vi "VI_get_version.vi"(8 "error in (no error)":errorcluster, 11 "vers block":string) -> (0 "error out":errorcluster, 3 "Version":T1 {"Flags" format="%04x"})   [LabVIEW 2023]
uses:
  <vilib>/Utility/error.llb/Error Cluster From Error Code.vi
  <vilib>/ErrorRing/Error Ring.xnode
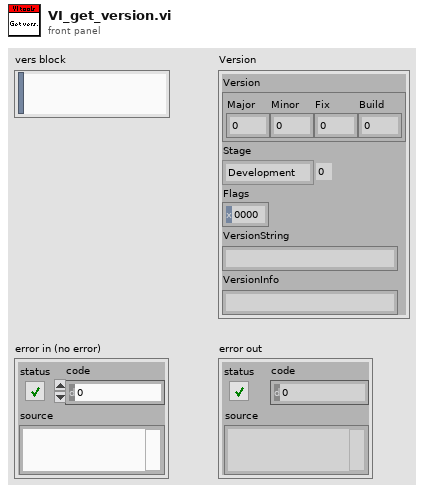
[diagram p1: front panel]
types:
  T1 = cluster{"Version":cluster{"Major":u8, "Minor":u8, "Fix":u8, "Build":u8}, "Stage":enum8{"Development", "Alpha", "Beta", "Release"}, "Flags":u16, "VersionString":string, "VersionInfo":string}
  T2 = cluster{"Version":u32, "Flags":u16, "VerStrLen":u8}
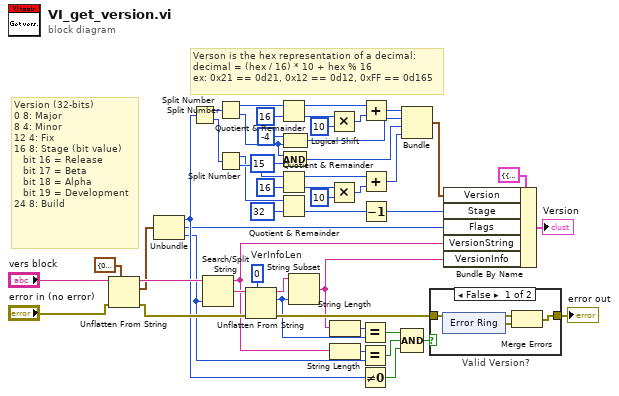
[diagram p0: block diagram]
diagram:
  w46 = u8 0  # VerInfoLen
  # "Verson is the hex representation of a decimal:\ndecimal = (hex / 16) * 10 + hex % 16\nex: 0x21 == 0d21, 0x12 == 0d12, 0xFF == 0d165"
  # "Version (32-bits)\n0 8: Major\n8 4: Minor\n12 4: Fix\n16 8: Stage (bit value)\n   bit 16 = Release\n   bit 17 = Beta\n   bit 18 = Alpha\n   bit 19 = Development\n24 8: Build"
  n1 = Unflatten From String(type=T2 {"Version"=0, "Flags"=0, "VerStrLen"=0} ("vers"), binary string="vers block", error in (no error)="error in (no error)") -> (rest of the binary string=w10:string, value=w4:T2, error out=w45:errorcluster)  [unwired: 2 in]
  n2 = Unbundle(w4) -> ("Version"=w3:u32, "Flags"=w2:u16, "VerStrLen"=w1:u8)
  n3 = Split Number(x=w3) -> (hi(x)=w42:u16, lo(x)=w43:u16)
  n4 = Search/Split String(string=w10, offset (0)=w1) -> (substring before match=w17:string, match + rest of string=w44:string)  [unwired: 1 in, 1 out]
  n5 = Split Number(x=w42) -> (hi(x)=w41:u8, lo(x)=w25:u8)
  n6 = Split Number(x=w43) -> (hi(x)=w21:u8, lo(x)=w30:u8)
  n7 = Unflatten From String(type=w46, binary string=w44, error in (no error)=w45) -> (rest of the binary string=w8:string, value=w9:u8, error out=w14:errorcluster)  [unwired: 2 in]
  n8 = Quotient & Remainder(x=w41, y=u8 16) -> (x-y*floor(x/y)=w36:u8, floor(x/y)=w39:u8)
  n9 = Quotient & Remainder(x=w30, y=u8 16) -> (x-y*floor(x/y)=w35:u8, floor(x/y)=w32:u8)
  n10 = Quotient & Remainder(x=w21, y=u8 32) -> (floor(x/y)=w20:u8)  [unwired: 1 out]
  n11 = Logical Shift(y=i16 -4, x=w25) -> (x << y=w23:u8)
  n12 = And(x=w25, y=u8 15) -> (x .and. y?=w26:u8)
  n13 = String Subset(string=w8, length (rest)=w9) -> (substring=w7:string)  [unwired: 1 in]
  n14 = Multiply(x=w39, y=u8 10) -> (x*y=w37:u8)
  n15 = Multiply(x=w32, y=u8 10) -> (x*y=w34:u8)
  n16 = String Length(string=w7) -> (length=w5:i32)
  n17 = String Length(string=w17) -> (length=w6:i32)
  n18 = Equal?(x=w5, y=w9) -> (x = y?=w16:bool)
  n19 = Equal?(x=w6, y=w1) -> (x = y?=w15:bool)
  n20 = Not Equal To 0?(x=w3) -> (x != 0?=w12:bool)
  n21 = Add(x=w36, y=w37) -> (x+y=w29:u8)
  n22 = Add(x=w35, y=w34) -> (x+y=w28:u8)
  n23 = Decrement(x=w20) -> (x-1=w18:u8)
  n24 = Compound Arithmetic op=AND(w16, w15, w12) -> (w13:bool)
  n25 = Bundle(w29, w23, w26, w28) -> (w19:cluster{u8, u8, u8, u8})  [unwired: 1 in]
  n26 = case "Valid Version?" shown="False" w13 {
    tunnel: [w53 w60] -> w49
    tunnel: w14 -> [w54 w60]
    frame False {
      n27 = xnode "Error Ring"() -> ("error out"=w52:errorcluster)
      n28 = Merge Errors(w54, w52) -> (w53:errorcluster)
    }
    frame True {
    }
  }
  "error out" <- w49
  n29 = Bundle By Name(cluster=T1 {"Version"={"Major"=0, "Minor"=0, "Fix"=0, "Build"=0}, "Stage"=enum."Development", "Flags"=0, "VersionString"="", "VersionInfo"=""} ("Version"), "Version"=w19, "Stage"=w18, "Flags"=w2, "VersionString"=w17, "VersionInfo"=w7) -> (→"Version":T1)
